vi "Write Var Map.vi"(8 "error in (no error)":errorcluster, 10 "Var Map":map{string, refnum<class "Abs_Type.lvclass">}(c390), 11 "Var Bus in":refnum<class "Multi_Bus.lvclass">) -> (0 "error out":errorcluster, 3 "Var Bus out":refnum<class "Multi_Bus.lvclass">)   [LabVIEW 2021, in "Multi_Bus.lvclass"]
uses:
  Multi_Bus.lvclass
  <vilib>/TSA/Abstract Data Classes/Abs_Types/Type/Abs_Type.lvclass
  Multi_Bus.lvclass/Multi_Bus.ctl
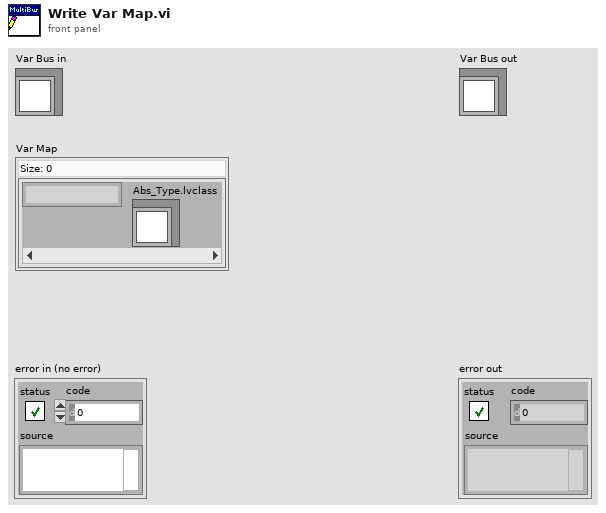
[diagram p1: front panel]
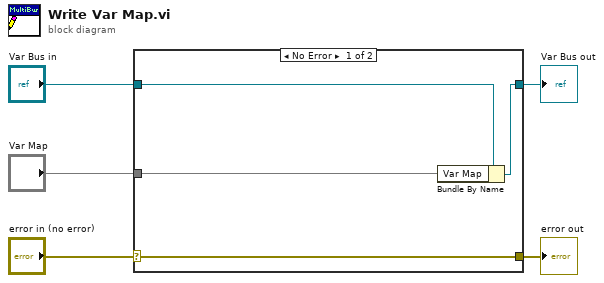
[diagram p0: block diagram]
diagram:
  n1 = case shown="No Error" "error in (no error)" {
    selector: "error in (no error)" -> [w9 w10]
    tunnel: [w9 w10] -> w4
    tunnel: [w7 w11] -> w2
    tunnel: "Var Bus in" -> [w8 w11]
    tunnel: "Var Map" -> [w6 _]
    frame No Error {
      n2 = Bundle By Name(cluster=w8, "Var Map"=w6) -> (w7:refnum<class "Multi_Bus.lvclass">)
    }
    frame Error {
    }
  }
  "error out" <- w4
  "Var Bus out" <- w2
